vi "Gait Event Detection Subvi.vi"(5 "Array":sgl[](array[numeric]), 7 "Threshold":dbl=0.15 min=0.0 max=5.0 step=0.05 format="%0.2f") -> (0 "Peak Indices":dbl[](array[numeric]), 1 "Uncorrected Peak Indices":dbl[](array[numeric]), 2 "Uncorrected Peak Duration":dbl[](array[numeric]), 3 "peak plot":cluster{dbl[], dbl[]}[](graph), 4 "True Peak Plot":cluster{"Ramp Pattern":dbl[], dbl[]}[](graph), 6 "Indices\nof False Peaks":dbl[](array[numeric]), 8 "Amplitudes at peak":dbl[](array[numeric]), 9 "Duplicate Indices\nof False Peaks":dbl[](array[numeric]), 10 "standard deviation":dbl format="%0.2f", 11 "Uncorrected Stance Duration":dbl format="%0.2f")   [LabVIEW 2011]
uses:
  <vilib>/Analysis/NI_AALBase.lvlib
  <vilib>/Analysis/1siggen.llb/Ramp Pattern by Samples.vi
  <vilib>/Analysis/NI_AALPro.lvlib
  <vilib>/Analysis/3filter.llb/Butterworth Filter (DBL).vi
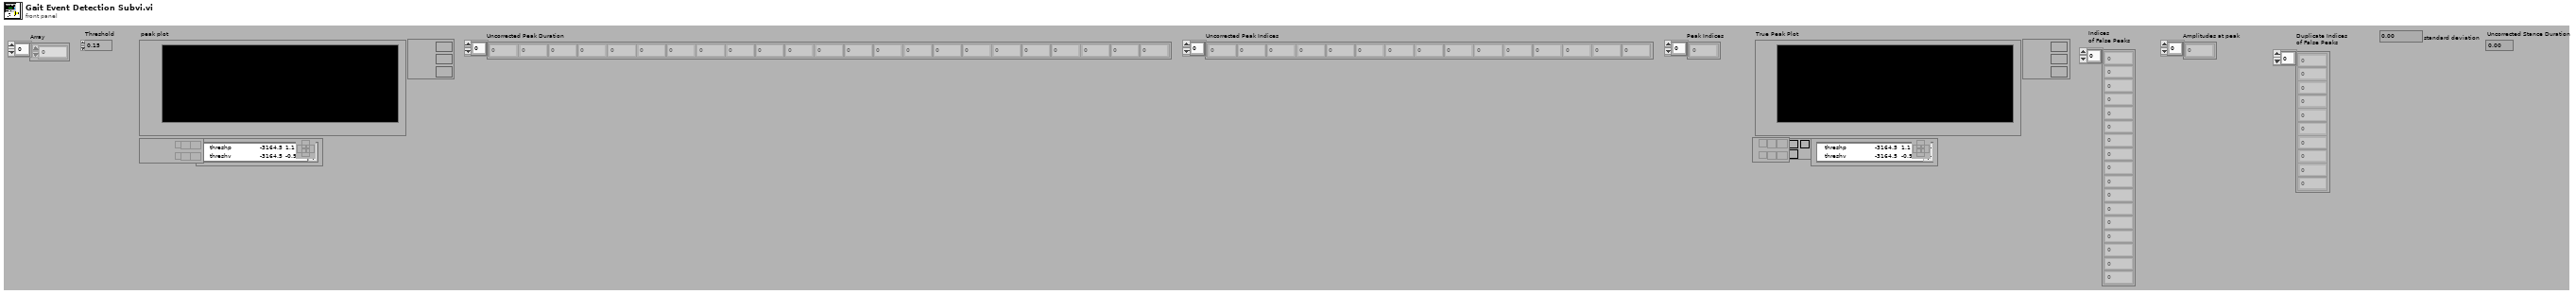
[diagram p1: front panel]
types:
  T1 = enum32{"Lowpass", "Highpass", "Bandpass", "Bandstop"}
  T2 = cluster{"Ramp Pattern":dbl[], "Amplitudes":dbl[]}[]
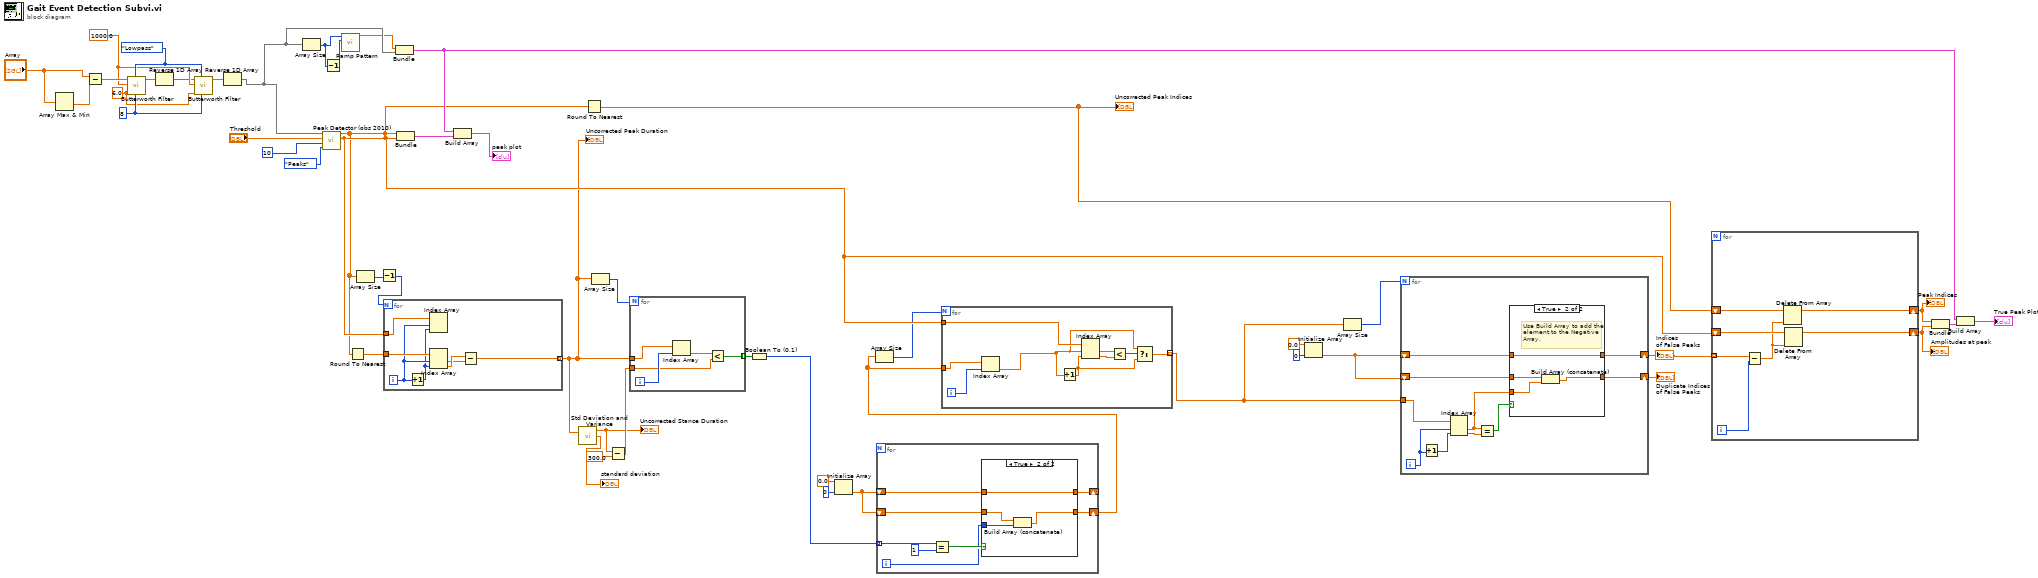
[diagram p0: block diagram]
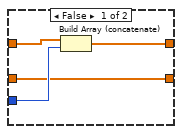
[diagram p2: hidden frame]
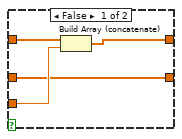
[diagram p3: hidden frame]
diagram:
  w16 = T1."Lowpass" ("filter type")
  w14 = 8 ("order")
  w12 = 1000.0 ("sampling freq: fs")
  w11 = 6.0 ("low cutoff freq: fl")
  n1 = Array Max & Min(array="Array") -> (min value=w17:sgl)  [unwired: 3 out]
  n2 = Subtract(x="Array", y=w17) -> (x-y=w19:sgl[])
  n3 = call-poly <vilib>:"Butterworth Filter.vi"("order"=w14, "filter type"=w16, "low cutoff freq: fl"=w11, "sampling freq: fs"=w12, "X"=w19) -> ("Filtered X"=w9:dbl[])  [unwired: 3 in, 1 out]
  n4 = Reverse 1D Array(array=w9) -> (reversed array=w10:dbl[])
  n5 = call-poly <vilib>:"Butterworth Filter.vi"("order"=w14, "filter type"=w16, "low cutoff freq: fl"=w11, "sampling freq: fs"=w12, "X"=w10) -> ("Filtered X"=w13:dbl[])  [unwired: 3 in, 1 out]
  n6 = Reverse 1D Array(array=w13) -> (reversed array=w15:dbl[])
  n7 = Array Size(array=w15) -> (size(s)=w4:i32)
  n8 = call <vilib>:"Peak Detector (obs 2010).vi"("peaks/valleys"=enum32{"Peaks", "Valleys"}."Peaks", "width"=10, "threshold"="Threshold", "X"=w15) -> ("Amplitudes"=w35:dbl[], "Locations"=w26:dbl[])  [unwired: 3 in, 3 out]
  n9 = Decrement(x=w4) -> (x-1=w5:i32)
  n10 = call-poly <vilib>:"Ramp Pattern.vi"("end"=w5, "samples"=w4) -> ("Ramp Pattern"=w6:dbl[])  [unwired: 8 in, 1 out]
  n11 = Round To Nearest(number=w26) -> (nearest integer value=w25:dbl[])
  n12 = Array Size(array=w26) -> (size(s)=w20:i32)
  n13 = Decrement(x=w20) -> (x-1=w21:i32)
  n14 = for {
    N: w21 -> [_]
    tunnel: w25 -> [w57]
    tunnel: [w51] -> w22 mode=indexing
    tunnel: w35 -> [w54]
    i -> [w53]
    n15 = Increment(x=w53) -> (x+1=w52:i32)
    n16 = Index Array(array=w54, index #1=w53, index #2=w52) -> ()  [unwired: 2 out]
    n17 = Index Array(array=w57, index #1=w53, index #2=w52) -> (element #1=w55:dbl, element #2=w56:dbl)
    n18 = Subtract(x=w56, y=w55) -> (x-y=w51:dbl)
  }
  "Uncorrected Peak Duration" <- w22
  n19 = Bundle("Ramp Pattern"=w6, w15) -> (w31:cluster{"Ramp Pattern":dbl[], dbl[]})  [unwired: 1 in]
  n20 = Bundle("Locations"=w26, "Amplitudes"=w35) -> (w8:cluster{"Locations":dbl[], "Amplitudes":dbl[]})  [unwired: 1 in]
  n21 = Build Array(w31, w8) -> (→"peak plot":cluster{"Locations":dbl[], "Amplitudes":dbl[]}[])
  n22 = call <vilib>:"Std Deviation and Variance.vi"("X"=w22) -> ("mean"=w28:dbl, "standard deviation"=→"standard deviation":dbl)  [unwired: 1 in, 1 out]
  "Uncorrected Stance Duration" <- w28
  n23 = Round To Nearest(number=w26) -> (nearest integer value=w34:dbl[])
  "Uncorrected Peak Indices" <- w34
  n24 = Array Size(array=w22) -> (size(s)=w24:i32)
  n25 = Subtract(x=w28, y=300.0) -> (x-y=w30:dbl)
  n26 = for {
    N: w24 -> [_]
    tunnel: w22 -> [w62]
    tunnel: w30 -> [w59]
    tunnel: [w58] -> w23 mode=indexing
    i -> [w61]
    n27 = Index Array(array=w62, index=w61) -> (element=w60:dbl)
    n28 = Less?(x=w60, y=w59) -> (x < y?=w58:bool)
  }
  n29 = Boolean To (0,1)(Boolean=w23) -> (0, 1=w46:i16[])
  n30 = Initialize Array(0.0, 0) -> (w49:dbl[])
  n31 = for {
    tunnel: w46 -> [w69] mode=indexing
    shift-right: [w64] -> _
    shift-left: w49 -> [w66]
    shift-right: [w63] -> w50
    shift-left: w49 -> [w65]
    i -> [w67]
    n32 = Equal?(x=w69, y=i16 1) -> (x = y?=w68:bool)
    n33 = case shown="True" w68 {
      tunnel: w67 -> [w72 w77]
      tunnel: [w73 w78] -> w64
      tunnel: w66 -> [w74 w78]
      tunnel: w65 -> [w71 w76]
      tunnel: [w71 w75] -> w63
      frame False {
        n34 = Build Array (concatenate)(w74, w72) -> (w73:dbl[])
      }
      frame True {
        n35 = Build Array (concatenate)(w76, w77) -> (w75:dbl[])
      }
    }
  }
  n36 = Array Size(array=w50) -> (size(s)=w27:i32)
  n37 = for {
    N: w27 -> [_]
    tunnel: w35 -> [w83]
    tunnel: [w82] -> w42 mode=indexing
    tunnel: w50 -> [w80]
    i -> [w81]
    n38 = Index Array(array=w80, index=w81) -> (element=w79:dbl)
    n39 = Increment(x=w79) -> (x+1=w87:dbl)
    n40 = Index Array(array=w83, index #1=w79, index #2=w87) -> (element #1=w85:dbl, element #2=w86:dbl)
    n41 = Less?(x=w85, y=w86) -> (x < y?=w84:bool)
    n42 = Select(t=w79, s=w84, f=w87) -> (s? t:f=w82:dbl)
  }
  n43 = Initialize Array(0.0, 0) -> (w41:dbl[])
  n44 = Array Size(array=w42) -> (size(s)=w44:i32)
  n45 = for {
    N: w44 -> [_]
    shift-right: [w97] -> w45
    shift-left: w41 -> [w96]
    shift-right: [w94] -> w43
    shift-left: w41 -> [w95]
    tunnel: w42 -> [w91]
    i -> [w92]
    n46 = Increment(x=w92) -> (x+1=w93:i32)
    n47 = Index Array(array=w91, index #1=w92, index #2=w93) -> (element #1=w89:dbl, element #2=w88:dbl)
    n48 = Equal?(x=w89, y=w88) -> (x = y?=w90:bool)
    n49 = case shown="True" w90 {
      tunnel: w89 -> [w99 w104]
      tunnel: [w100 w105] -> w97
      tunnel: w96 -> [w101 w105]
      tunnel: w95 -> [w98 w103]
      tunnel: [w98 w102] -> w94
      frame False {
        n50 = Build Array (concatenate)(w101, w99) -> (w100:dbl[])
      }
      frame True {
        # "Use Build Array to add the\nelement to the Negative\nArray."
        n51 = Build Array (concatenate)(w103, w104) -> (w102:dbl[])
      }
    }
  }
  "Indices\nof False Peaks" <- w45
  "Duplicate Indices\nof False Peaks" <- w43
  n52 = for {
    shift-right: [w107] -> w36
    shift-left: w34 -> [w112]
    shift-right: [w106] -> w37
    shift-left: w35 -> [w109]
    tunnel: w45 -> [w111] mode=indexing
    i -> [w110]
    n53 = Subtract(x=w111, y=w110) -> (x-y=w108:dbl)
    n54 = Delete From Array(array=w112, index=w108) -> (array with subset deleted=w107:dbl[])  [unwired: 1 in, 1 out]
    n55 = Delete From Array(array=w109, index=w108) -> (array with subset deleted=w106:dbl[])  [unwired: 1 in, 1 out]
  }
  "Peak Indices" <- w36
  "Amplitudes at peak" <- w37
  n56 = Bundle(w36, "Amplitudes"=w37) -> (w38:cluster{dbl[], "Amplitudes":dbl[]})  [unwired: 1 in]
  n57 = Build Array(w31, w38) -> (→"True Peak Plot":T2)
